vi "Decrement.vi"(8 "error in (no error)":errorcluster, 11 "Contador in":refnum<class "Contador.lvclass">) -> (0 "error out":errorcluster, 3 "Contador out":refnum<class "Contador.lvclass">)   [LabVIEW 2020, in "Contador.lvlib" / "Contador.lvclass"]
uses:
  Contador.lvclass
  Contador.lvclass/Contador.ctl
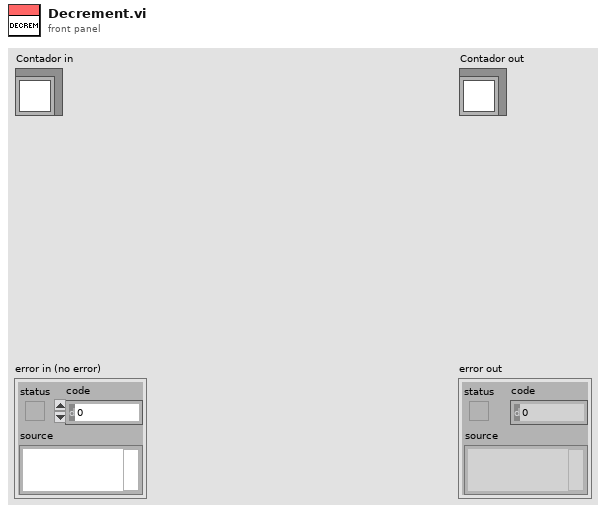
[diagram p1: front panel]
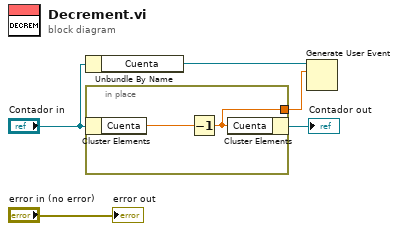
[diagram p0: block diagram]
diagram:
  n1 = Unbundle By Name("Contador in") -> ("Cuenta"=w2:refnum<user-event>)
  n2 = in-place {
    in-place-border: [w6] -> w1
    n3 = in-place-cluster #1("Contador in") -> ("Cuenta"=w7:dbl)
    n4 = Decrement(x=w7) -> (x-1=w6:dbl)
    n5 = in-place-cluster #1("Cuenta"=w6) -> (→"Contador out":refnum<class "Contador.lvclass">)
  }
  n6 = Generate User Event(user event=w2, event data cluster=w1) -> ()  [unwired: 2 in, 2 out]
  "error out" <- "error in (no error)"
